vi "lib_path_mod_20200519.vi"() -> (2 "path":path)   [LabVIEW 2018]
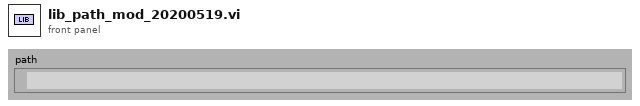
[diagram p1: front panel]
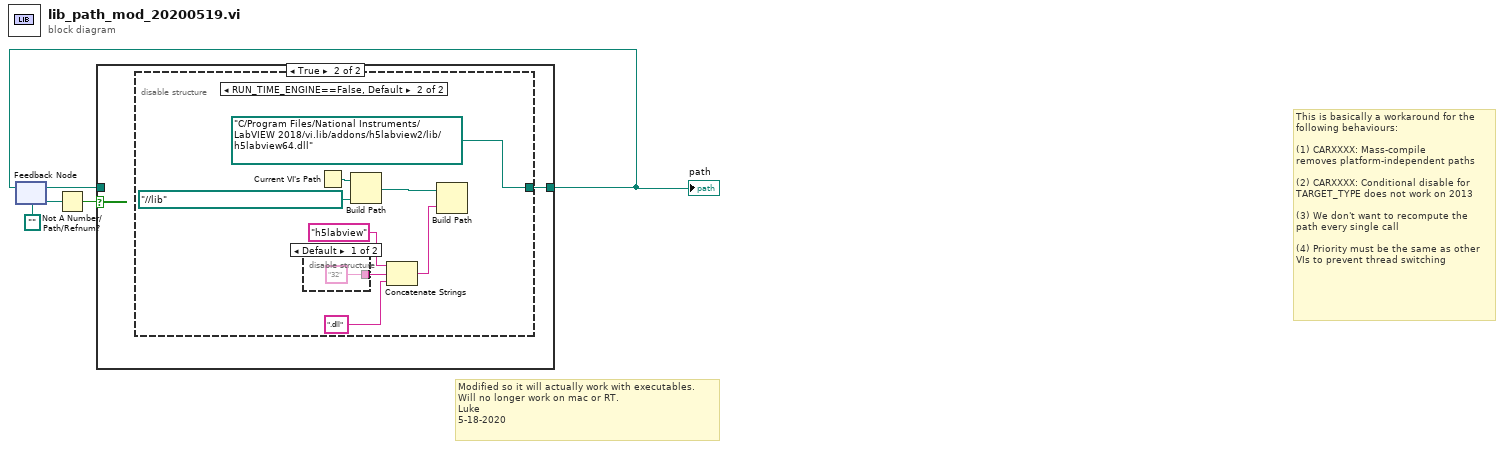
[diagram p0: block diagram]
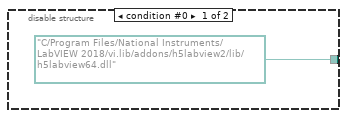
[diagram p3: hidden frame]
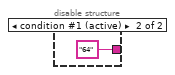
[diagram p4: hidden frame]
diagram:
  # "Modified so it will actually work with executables.\nWill no longer work on mac or RT.\nLuke \n5-18-2020"
  # "This is basically a workaround for the\nfollowing behaviours:\n\n(1) CARXXXX: Mass-compile\nremoves platform-independent paths\n\n(2) CARXXXX: Conditional disable for\nTARGET_TYPE does not work on 2013\n\n(3) We don't want to recompute the\npath every single call\n\n(4) Priority must be the same as other\nVIs to prevent thread switching"
  n1 = feedback #1(path "") -> (w2:path)
  n2 = Not A Number/Path/Refnum?(number/path/refnum=w2) -> (NaN/Path/Refnum?=w3:bool)
  n3 = case shown="True" w3 {
    tunnel: w2 -> [w5 _]
    tunnel: [w5 w6] -> w1
    frame False {
    }
    frame True {
      n4 = disable-structure shown="RUN_TIME_ENGINE==False, Default" {
        disable-tunnel: [path "C:/Program Files/National Instruments/LabVIEW 2018/vi.lib/addons/h5labview2/lib/h5labview64.dll" ("path") path "C:/Program Files/National Instruments/LabVIEW 2018/vi.lib/addons/h5labview2/lib/h5labview64.dll" ("path")] -> w6
        frame condition #0 {
        }
        frame condition #1 (active) {
          n5 = disable-structure shown="Default" {
            disable-tunnel: ["32" "64"] -> w13
            frame condition #0 {
            }
            frame condition #1 (active) {
            }
          }
          n6 = Current VI's Path() -> (path=w15:path)
          n7 = Build Path(base path=w15, name or relative path=path "../../lib" ("appended path")) -> (appended path=w12:path)
          n8 = Concatenate Strings("h5labview", w13, ".dll") -> (w14:string)
          n9 = Build Path(base path=w12, name or relative path=w14) -> ()  [unwired: 1 out]
        }
      }
    }
  }
  "path" <- w1
  n10 = feedback-in #1(w1) -> ()
